vi "Initialize.vi"(8 "error in (no error)":errorcluster, 10 "Top Level Diagram":refnum<vi>, 11 "IO Loop in":refnum<class "Module Loop.lvclass">) -> (0 "error out":errorcluster, 3 "IO Loop out":refnum<class "Module Loop.lvclass">)   [LabVIEW 2025, in "Module Loop.lvclass"]
uses:
  Module Loop.lvclass
  Structures/Structures.lvclass/Structures.ctl
  <vilib>/Utility/miscctls.llb/LVPointTypeDef.ctl
  Loop/Loop.lvclass/Loop.ctl
  Loop/Write Loop Structure.vi
  Structures/Read Name.vi
  Structures/Write Location.vi
  Structures/Structures.lvclass
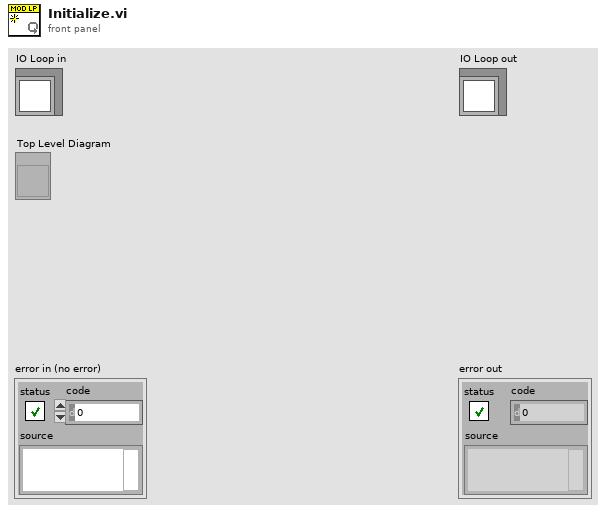
[diagram p1: front panel]
types:
  T1 = typedef "LVPointTypeDef.ctl" = cluster{"Horizontal":i16, "Vertical":i16}
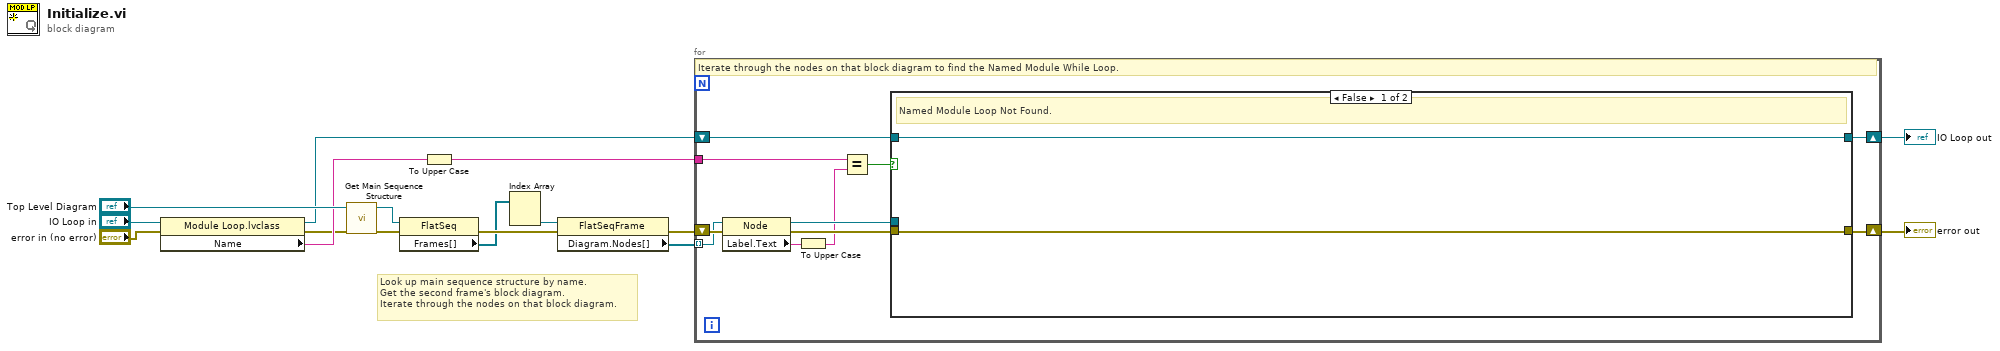
[diagram p0: block diagram]
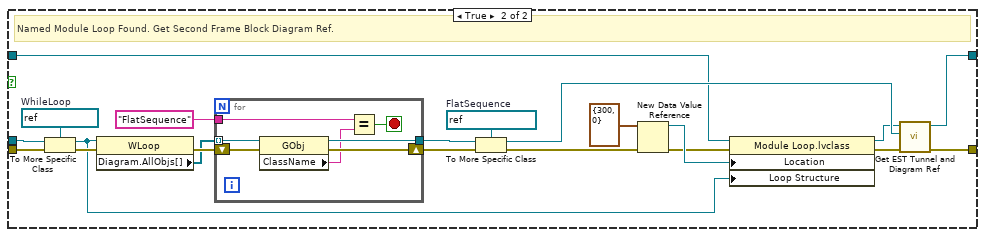
[diagram p2: hidden frame]
diagram:
  # "Look up main sequence structure by name.\nGet the second frame's block diagram.\nIterate through the nodes on that block diagram."
  n1 = property class="Module Loop.lvclass"(reference="IO Loop in", error in="error in (no error)") -> (reference out=w2:refnum<class "Module Loop.lvclass">, error out=w1:errorcluster, "Name"=w4:string)
  n2 = call "Get Main Sequence Structure.vi"("error in (no error)"=w1, "Top Level Diagram"="Top Level Diagram") -> ("error out"=w9:errorcluster, "Main.SeqStructure"=w8:refnum<vi>)  [unwired: 8 in]
  n3 = property class="FlatSeq"(reference=w8, error in=w9) -> (error out=w13:errorcluster, "Frames[]"=w12:refnum<vi>[])  [unwired: 1 out]
  n4 = To Upper Case(1:w4) -> (0:w11:string)
  n5 = Index Array(array=w12) -> (element #2=w16:refnum<vi>)  [unwired: 2 in, 1 out]
  n6 = property class="FlatSeqFrame"(reference=w16, error in=w13) -> (error out=w15:errorcluster, "Diagram.Nodes[]"=w14:refnum<vi>[])  [unwired: 1 out]
  n7 = for {
    tunnel: w14 -> [w26] mode=indexing
    shift-right: [w22] -> w10
    shift-left: w15 -> [w27]
    tunnel: w11 -> [w20]
    shift-right: [w18] -> w6
    shift-left: w2 -> [w19]
    # "Iterate through the nodes on that block diagram to find the Named Module While Loop."
    n8 = property class="Node"(reference=w26, error in=w27) -> (reference out=w24:refnum<vi>, error out=w23:errorcluster, "Label.Text"=w25:string)
    n9 = To Upper Case(1:w25) -> (0:w21:string)
    n10 = Equal?(x=w20, y=w21) -> (x = y?=w17:bool)
    n11 = case shown="False" w17 {
      tunnel: w24 -> [_ w49]
      tunnel: w23 -> [w29 w50]
      tunnel: [w29 w39] -> w22
      tunnel: w19 -> [w28 w37]
      tunnel: [w28 w38] -> w18
      frame False {
        # "Named Module Loop Not Found."
      }
      frame True {
        w48 = refnum<vi> refnum  # WhileLoop
        w43 = refnum<vi> refnum  # FlatSequence
        # "Named Module Loop Found. Get Second Frame Block Diagram Ref."
        n12 = To More Specific Class(target class=w48, reference=w49, error in=w50) -> (specific class reference=w34:refnum<vi>, error out=w47:errorcluster)
        n13 = property class="WLoop"(reference=w34, error in=w47) -> (error out=w46:errorcluster, "Diagram.AllObjs[]"=w45:refnum<vi>[])  [unwired: 1 out]
        n14 = for {
          shift-right: [w56] -> w44
          shift-left: w46 -> [w57]
          tunnel: w45 -> [w55] mode=indexing
          tunnel: "FlatSequence" ("name/order") -> [w54]
          tunnel: [w52] -> w41
          stop <- w53 stop-if-true
          n15 = property class="GObj"(reference=w55, error in=w57) -> (reference out=w52:refnum<vi>, error out=w56:errorcluster, "ClassName"=w51:string)
          n16 = Equal?(x=w54, y=w51) -> (x = y?=w53:bool)
        }
        n17 = To More Specific Class(target class=w43, reference=w41, error in=w44) -> (specific class reference=w40:refnum<vi>, error out=w31:errorcluster)
        n18 = New Data Value Reference(data value=T1 {"Horizontal"=300, "Vertical"=0} ("location out"), error in=w31) -> (data value reference=w32:refnum<data-value>, error out=w30:errorcluster)
        n19 = property class="Module Loop.lvclass"(reference=w37, error in=w30, "Location"=w32, "Loop Structure"=w34) -> (reference out=w36:refnum<class "Module Loop.lvclass">, error out=w35:errorcluster)
        n20 = call-dynamic "Get EST Tunnel and Diagram Ref.vi"("error in (no error)"=w35, "FlatSeq Refnum"=w40, "IO Loop in"=w36) -> ("error out"=w39:errorcluster, "IO Loop out"=w38:refnum<class "Module Loop.lvclass">)  [unwired: 7 in]
      }
    }
  }
  "error out" <- w10
  "IO Loop out" <- w6
